vi "NML Wait Until Next ms Multiple.vi"(11 "Delay (mS)":u32) -> (3 "Timestamp":dbl format="%_16f")   [LabVIEW 2021]
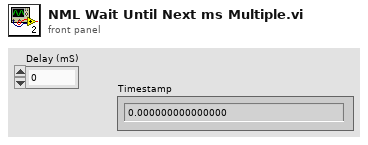
[diagram p1: front panel]
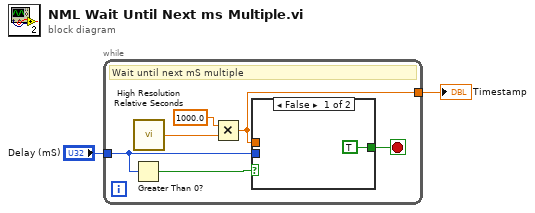
[diagram p0: block diagram]
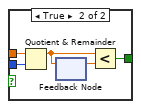
[diagram p2: hidden frame]
diagram:
  n1 = while {
    tunnel: "Delay (mS)" -> [w3]
    tunnel: [w6] -> w1
    stop <- w5 stop-if-true
    # "Wait until next mS multiple"
    n2 = Greater Than 0?(x=w3) -> (x > 0?=w4:bool)
    n3 = call <vilib>:"High Resolution Relative Seconds.vi"() -> ("relative seconds"=w8:dbl)
    n4 = Multiply(x=1000.0, y=w8) -> (x*y=w6:dbl)
    n5 = case shown="False" w4 {
      tunnel: w3 -> [_ w14]
      tunnel: w6 -> [_ w13]
      tunnel: [TRUE w10] -> w5
      frame False {
      }
      frame True {
        n6 = Quotient & Remainder(x=w13, y=w14) -> (x-y*floor(x/y)=w11:dbl)  [unwired: 1 out]
        n7 = feedback #1() -> (w12:dbl)  [unwired: 1 in]
        n8 = feedback-in #1(w11) -> ()
        n9 = Less?(x=w11, y=w12) -> (x < y?=w10:bool)
      }
    }
  }
  "Timestamp" <- w1
